vi "Periodic Tasks.vi"(8 "error in":errorcluster) -> ()   [LabVIEW 2016]
doc: "This VI runs in parallel to other tasks. It can contain as many user-defined periodic loops as you need. These can carry out PID or other sorts of timed response."
uses:
  <vilib>/Rock Robotics/WPI/DriverStation/WPI_DriverStationRobotMode2.ctl
  Robot Global Data.vi
  <vilib>/Rock Robotics/Network Tables/NT Write Boolean.vi
  <vilib>/Rock Robotics/Network Tables/NT Write Number.vi
  <vilib>/Rock Robotics/Network Tables/NT Read String.vi
  <vilib>/Rock Robotics/Network Tables/NT Write String.vi
  <vilib>/Rock Robotics/Network Tables/NT Read Number.vi
  <vilib>/Rock Robotics/WPI/Utilities/WPI_GetSetVariantRefNum.vi
  <vilib>/Rock Robotics/Network Tables/NT Read Numeric Array.vi
  <vilib>/Rock Robotics/Network Tables/NT Read Boolean.vi
  <vilib>/Rock Robotics/Network Tables/NT Write Numeric Array.vi
panel:
  in  "milliseconds to wait":u32=20
  out "Averaged Values 2":dbl(graph)
  out "Channel 1":dbl(graph)
  out "Channel 0":dbl(graph)
  in  "Range":dbl=100.0 format="%#_13g"
  out "Averaged Values":dbl(graph)=25.833333333333332
  out "<5?":i16(graph)=1
  out "Image Width":dbl(graph)=26.0
  in  "Past array Width":dbl[](array[numeric])=[26.0, 26.0, 26.0, 25.0, 26.0, 26.0]
  out "Gear Orient":bool=TRUE
  out "Gear In":bool=TRUE
  out "1 Width":dbl=17.0
  out "1 Height":dbl=26.0
  out "2 Width":dbl=8.5
  out "2 Height":dbl=13.0
  in  "Past array":dbl[](array[numeric])=[-10.0, -10.0, -10.0]
  in  "Lcal Pixy Out":dbl=-10.0
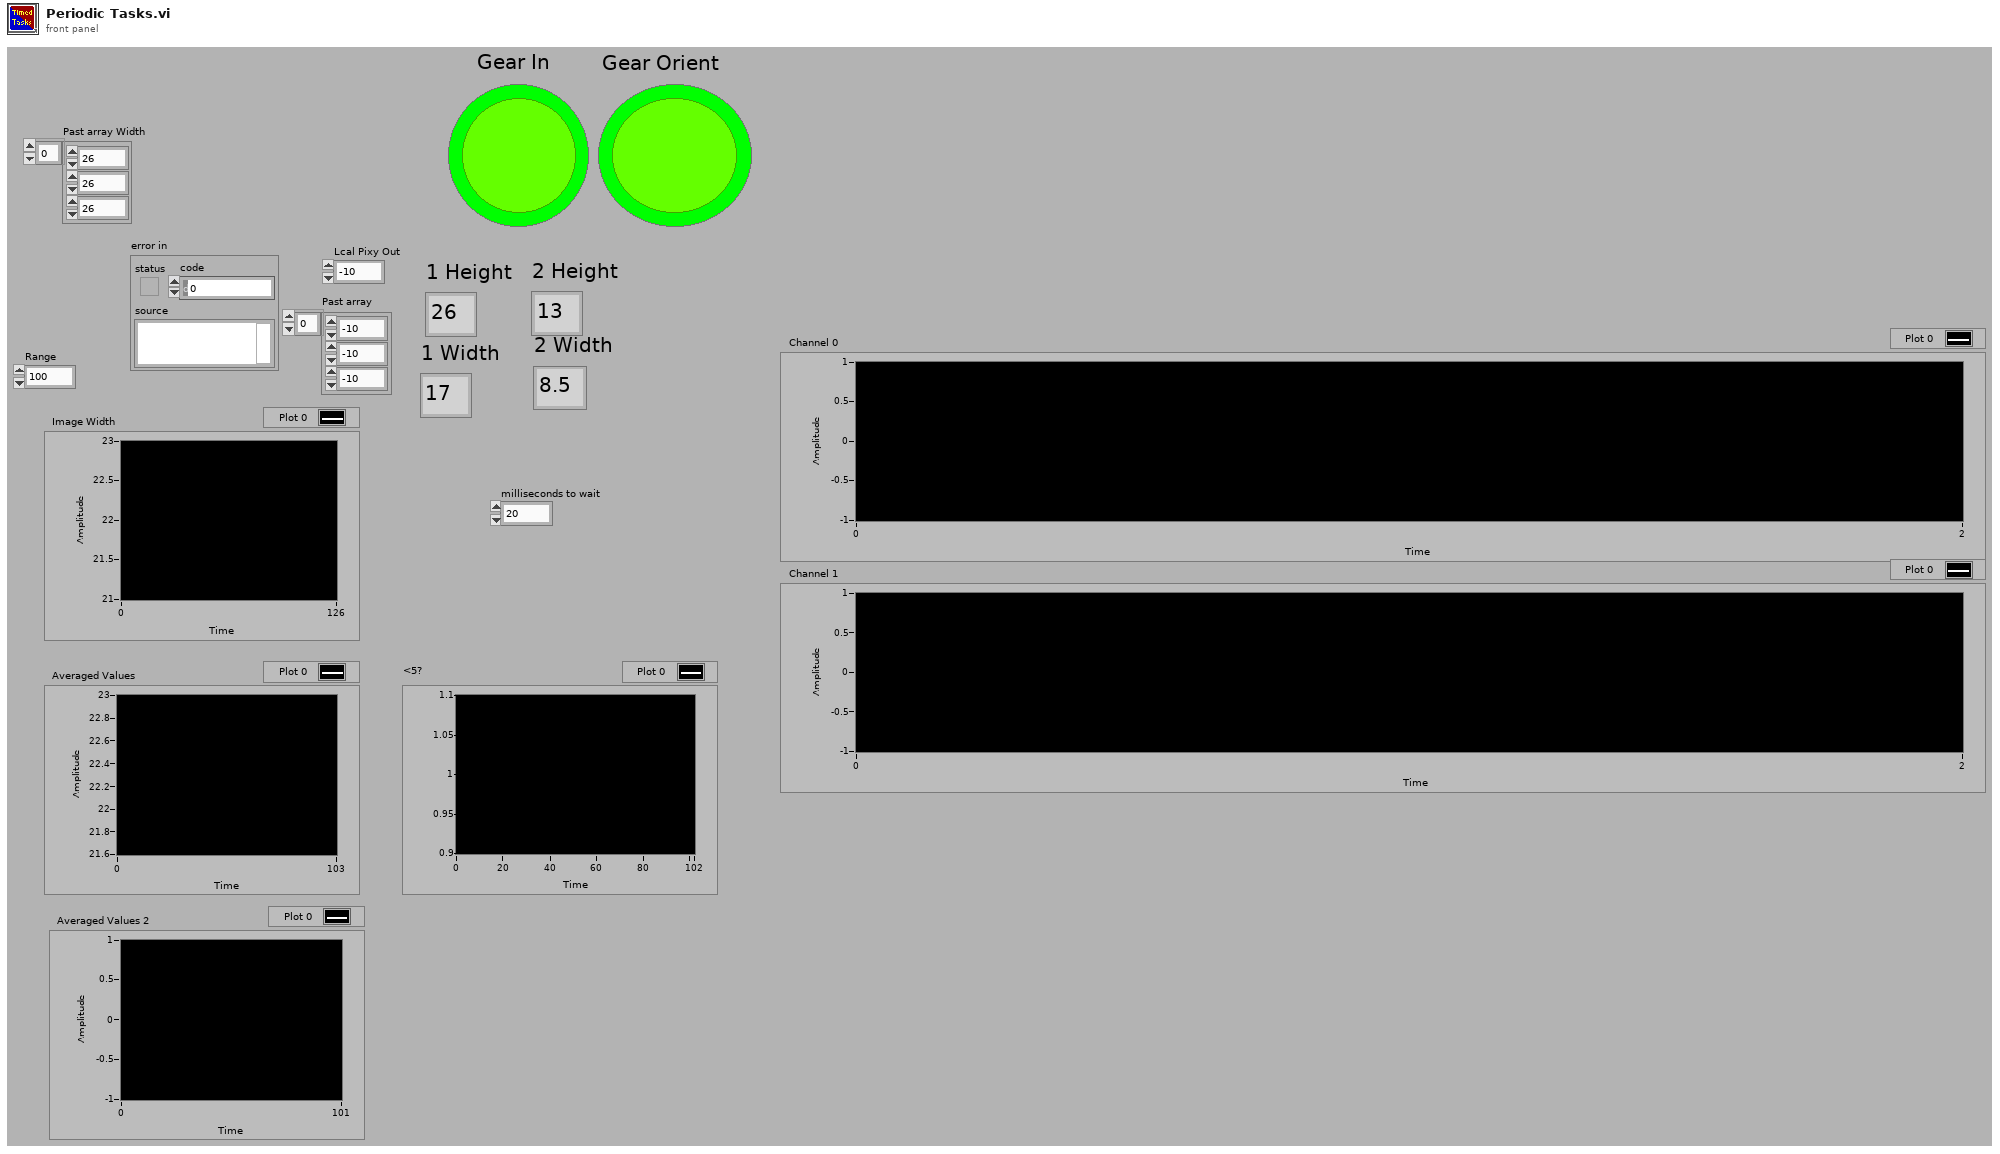
[diagram p1: front panel]
types:
  T1 = typedef "WPI_SwitchDevRef.ctl" = cluster{"DevStatus":errorcluster, "DIO Channel":T2, "CntIndex":T3, "Normally Closed":bool}
  T2 = typedef "FPGA_DIOChannel.ctl" = enum8{"DIO 0", "DIO 1", "DIO 2", "DIO 3", "DIO 4", "DIO 5", "DIO 6", "DIO 7", "DIO 8", "DIO 9", "DIO MXP 0", "DIO MXP 1", "DIO MXP 2", "DIO MXP 3", "DIO MXP 4", "DIO MXP 5", "DIO MXP 6", "DIO MXP 7", "DIO MXP 8", "DIO MXP 9", "DIO MXP 10", "DIO MXP 11", "DIO MXP 12", "DIO MXP 13", "DIO MXP 14", "DIO MXP 15", "SPI Port CS1", "SPI Port CS2", "SPI Port CS3", "SPI Port MISO", "SPI Port MOSI", "Invalid"}
  T3 = typedef "FPGA_CounterCtrSystemIndex.ctl" = enum8{"Ctr 0", "Ctr 1", "Ctr 2", "Ctr 3", "Ctr 4", "Ctr 5", "Ctr 6", "Ctr 7", "Invalid"}
  T4 = typedef "WPI_ServoDeviceRef.ctl" = cluster{"DeviceStatus":errorcluster, "PWM Channel":T5, "DeadBand":T6}
  T5 = typedef "FPGA_DIOPWMChannel.ctl" = enum8{"PWM 0", "PWM 1", "PWM 2", "PWM 3", "PWM 4", "PWM 5", "PWM 6", "PWM 7", "PWM 8", "PWM 9", "PWM MXP 0", "PWM MXP 1", "PWM MXP 2", "PWM MXP 3", "PWM MXP 4", "PWM MXP 5", "PWM MXP 6", "PWM MXP 7", "PWM MXP 8", "PWM MXP 9", "Invalid"}
  T6 = typedef "WPI_PWMDeadband.ctl" = cluster{"Name":string, "maxPositivePwm":i32, "minPositivePwm":i32, "centerPwm":i32, "maxNegativePwm":i32, "minNegativePwm":i32, "angularRange":u16}
  T7 = typedef "WPI_CounterDevRef.ctl" = cluster{"DevStatus":errorcluster, "CntIndex":T3}
  T8 = typedef "WPI_JoystickDevRef.ctl" = cluster{"Device":T9}
  T9 = typedef "WPI_JoystickDeviceEnum.ctl" = enum16{"USB 0", "USB 1", "USB 2", "USB 3", "USB 4", "USB 5"}
  T10 = typedef "WPI_DriverStationRobotMode2.ctl" = enum16{"Autonomous Disabled", "Autonomous Enabled", "Teleop Disabled", "Teleop Enabled", "Disconnected", "Finish", "Test Disabled", "Test Enabled", "Emergency Stopped"}
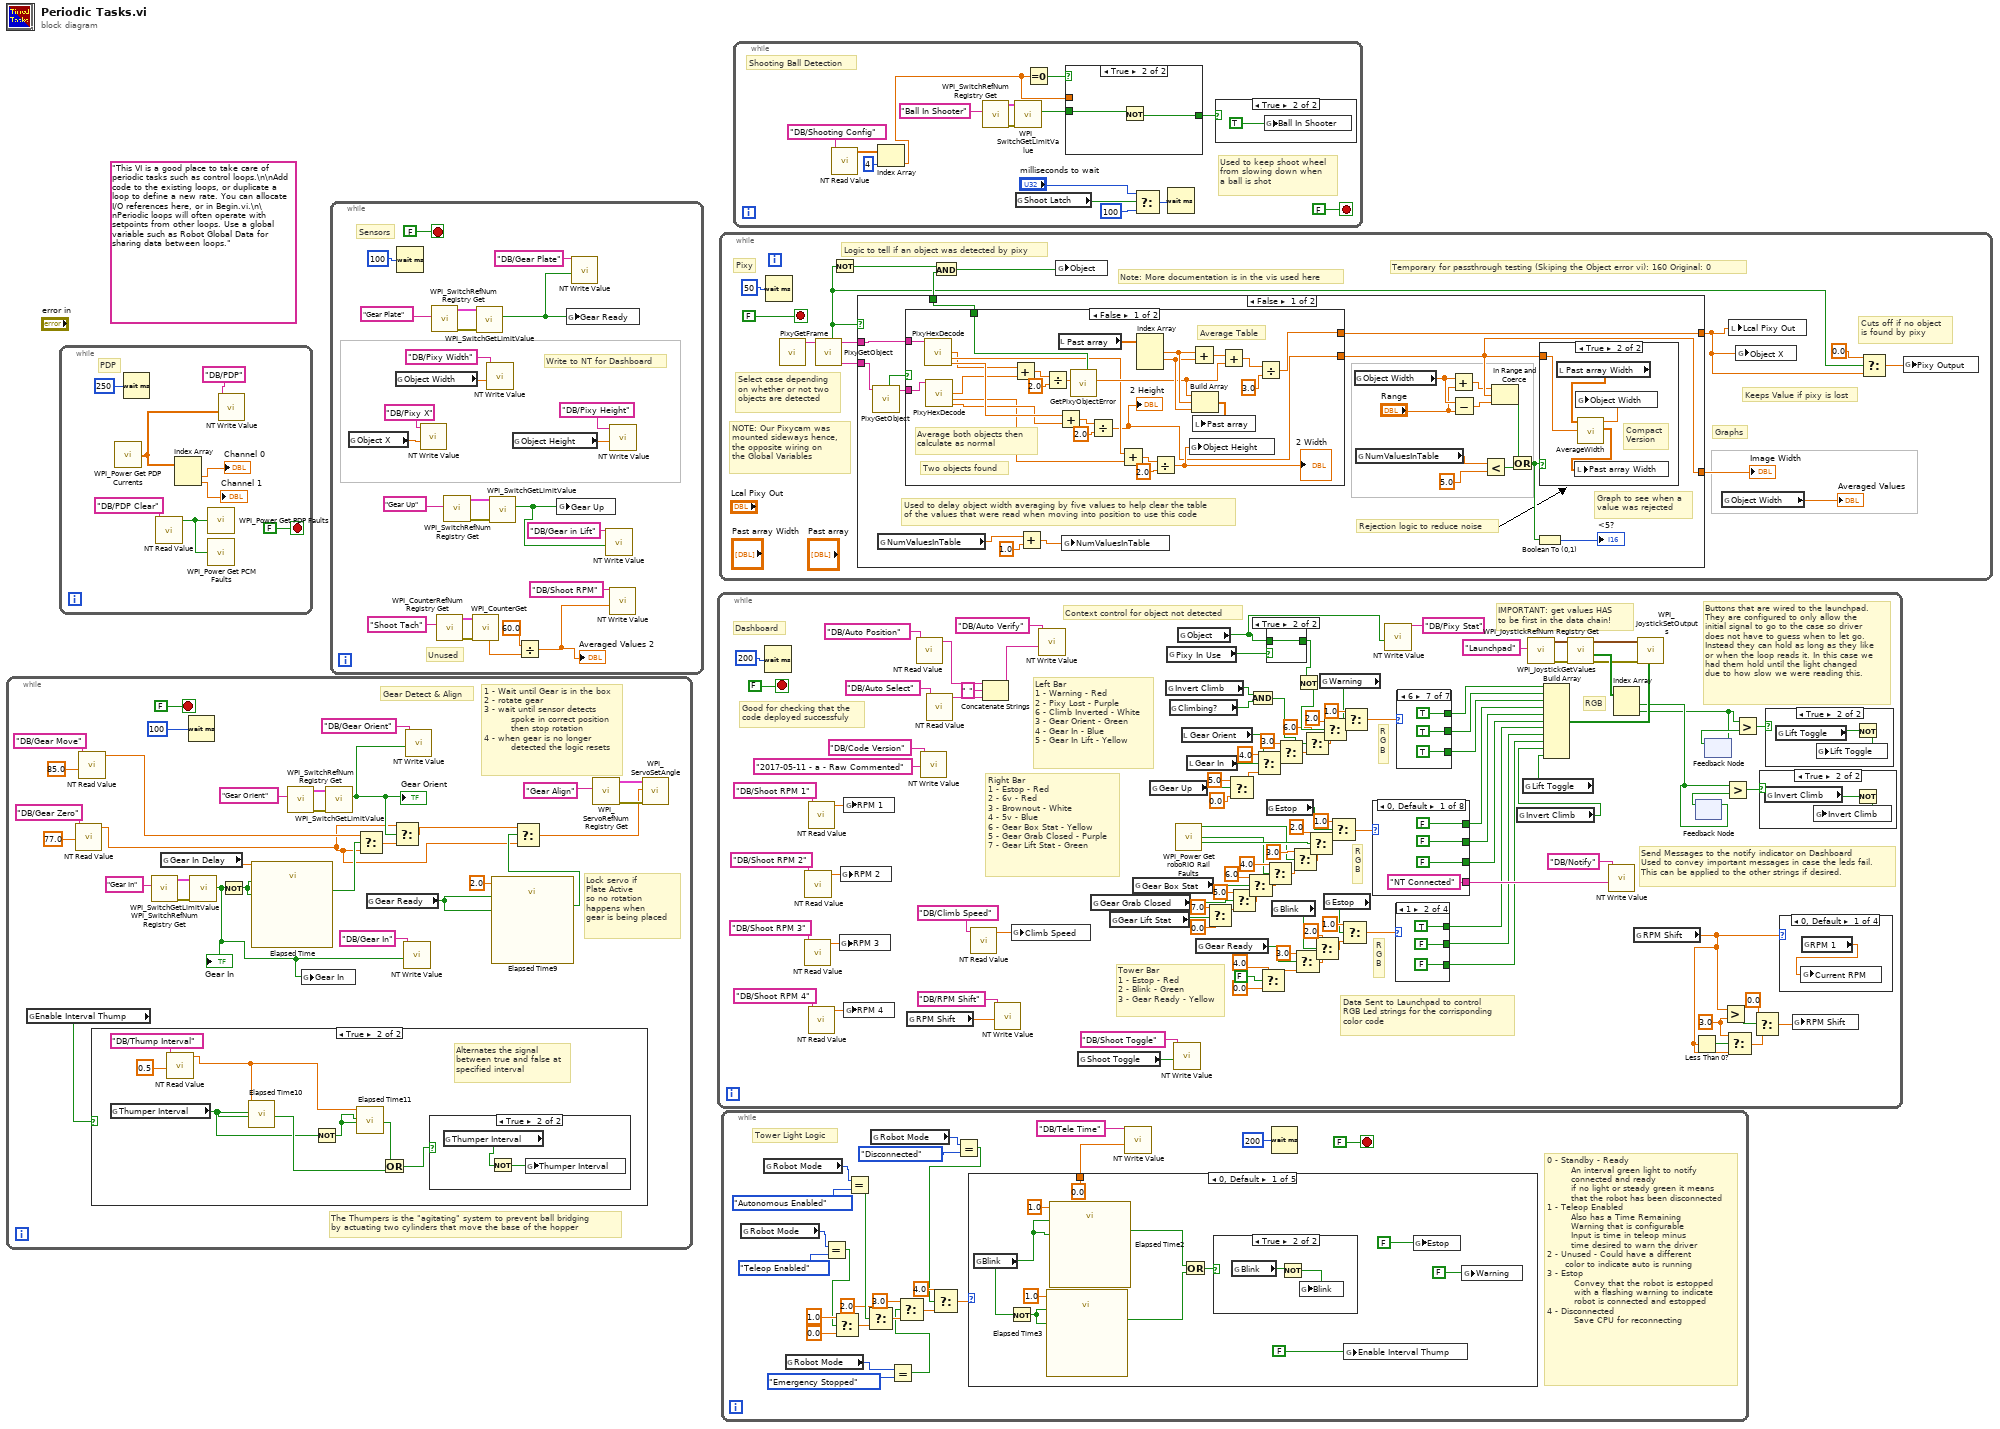
[diagram p0: block diagram]
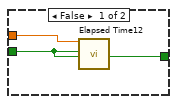
[diagram p2: hidden frame]
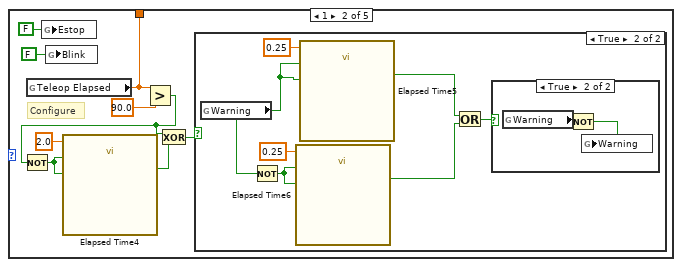
[diagram p5: hidden frame]
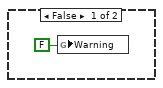
[diagram p6: hidden frame]
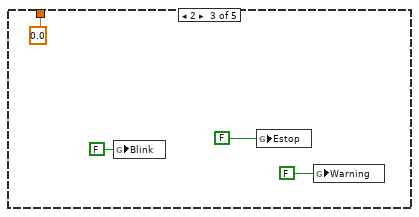
[diagram p8: hidden frame]
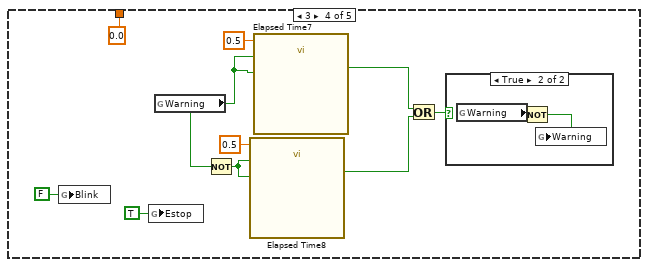
[diagram p9: hidden frame]
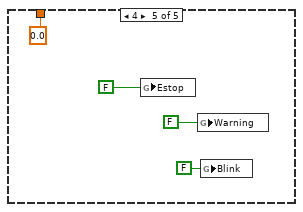
[diagram p11: hidden frame]
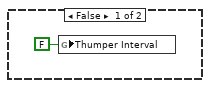
[diagram p12: hidden frame]
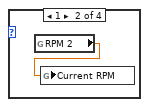
[diagram p14: hidden frame]
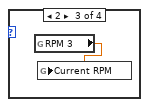
[diagram p15: hidden frame]
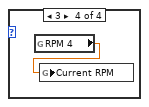
[diagram p16: hidden frame]
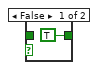
[diagram p19: hidden frame]
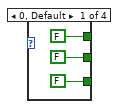
[diagram p20: hidden frame]
diagram:
  (unwired) "This VI is a good place to take care of periodic tasks such as control loops.\n\nAdd code to the existing loops, or duplicate a loop to define a new rate. You can allocate I/O references here, or in Begin.vi.\n\nPeriodic loops will often operate with setpoints from other loops. Use a global variable such as Robot Global Data for sharing data between loops."
  n1 = while {
    stop <- FALSE stop-if-true
    # "1 - Wait until Gear is in the box\n2 - rotate gear \n3 - wait until sensor detects \n         spoke in correct position\n         then stop rotation\n4 - when gear is no longer \n         detected the logic resets"
    # "The Thumpers is the \"agitating\" system to prevent ball bridging \nby actuating two cylinders that move the base of the hopper"
    # "Lock servo if\nPlate Active\nso no rotation\nhappens when\ngear is being placed"
    # "Gear Detect & Align"
    n2 = global read "Robot Global Data.vi" "Enable Interval Thump"() -> (w1:bool)
    n3 = call-poly <vilib>:"NT Read Value.vi"("Default Value"=77.0, "Name"="DB/Gear Zero") -> ("Numeric"=w3:dbl)  [unwired: 8 in, 1 out]
    n4 = call-poly <vilib>:"NT Read Value.vi"("Default Value"=85.0, "Name"="DB/Gear Move") -> ("Numeric"=w11:dbl)  [unwired: 8 in, 1 out]
    n5 = case shown="True" w1 {
      frame False {
        n6 = global write "Robot Global Data.vi" "Thumper Interval"(FALSE ("Thumper Interval")) -> ()
      }
      frame True {
        # "Alternates the signal\nbetween true and false at\nspecified interval"
        n7 = global read "Robot Global Data.vi" "Thumper Interval"() -> (w36:bool)
        n8 = call-poly <vilib>:"NT Read Value.vi"("Default Value"=0.5, "Name"="DB/Thump Interval") -> ("Numeric"=w33:dbl)  [unwired: 8 in, 1 out]
        n9 = call "Elapsed Time10"("Time Target (s)"=w33, "Reset"=w36, "Auto Reset"=w36) -> ("Time has Elapsed"=w38:bool)  [unwired: 9 in, 7 out]
        n10 = Not(x=w36) -> (.not. x?=w40:bool)
        n11 = call "Elapsed Time11"("Time Target (s)"=w33, "Reset"=w40, "Auto Reset"=w40) -> ("Time has Elapsed"=w39:bool)  [unwired: 9 in, 7 out]
        n12 = Or(x=w39, y=w38) -> (x .or. y?=w37:bool)
        n13 = case shown="True" w37 {
          frame False {
          }
          frame True {
            n14 = global read "Robot Global Data.vi" "Thumper Interval"() -> (w42:bool)
            n15 = Not(x=w42) -> (.not. x?=w41:bool)
            n16 = global write "Robot Global Data.vi" "Thumper Interval"(w41) -> ()
          }
        }
      }
    }
    n17 = call <vilib>:"WPI_SwitchRefNum Registry Get.vi"("refnum name"="Gear In") -> ("error out"=w28:errorcluster, "SwitchDevRef"=w29:T1)  [unwired: 9 in]
    n18 = global read "Robot Global Data.vi" "Gear In Delay"() -> (w21:dbl)
    n19 = Wait (ms)(milliseconds to wait=u32 100) -> ()  [unwired: 1 out]
    n20 = call <vilib>:"WPI_SwitchGetLimitValue.vi"("error in (no error)"=w28, "SwitchDevRef"=w29) -> ("Switch Pressed"=w2:bool)  [unwired: 7 in, 2 out]
    "Gear In" <- w2
    n21 = Not(x=w2) -> (.not. x?=w22:bool)
    n22 = call "Elapsed Time"("Time Target (s)"=w21, "Reset"=w22, "Auto Reset"=w22) -> ("Time has Elapsed"=w16:bool)  [unwired: 9 in, 7 out]
    n23 = call <vilib>:"WPI_SwitchRefNum Registry Get.vi"("refnum name"="Gear Orient") -> ("error out"=w24:errorcluster, "SwitchDevRef"=w25:T1)  [unwired: 9 in]
    n24 = global write "Robot Global Data.vi" "Gear In"(w2) -> ()
    n25 = call <vilib>:"WPI_SwitchGetLimitValue.vi"("error in (no error)"=w24, "SwitchDevRef"=w25) -> ("Switch Pressed"=w14:bool)  [unwired: 7 in, 2 out]
    "Gear Orient" <- w14
    n26 = Select(t=w11, s=w16, f=w3) -> (s? t:f=w26:dbl)
    n27 = global read "Robot Global Data.vi" "Gear Ready"() -> (w7:bool)
    n28 = Select(t=w3, s=w14, f=w26) -> (s? t:f=w4:dbl)
    n29 = call-poly <vilib>:"NT Write Value.vi"("Boolean"=w2, "Name"="DB/Gear In") -> ()  [unwired: 9 in, 1 out]
    n30 = call-poly <vilib>:"NT Write Value.vi"("Boolean"=w14, "Name"="DB/Gear Orient") -> ()  [unwired: 9 in, 1 out]
    n31 = call "Elapsed Time9"("Time Target (s)"=2.0, "Reset"=w7, "Auto Reset"=w7) -> ("Time has Elapsed"=w5:bool)  [unwired: 9 in, 7 out]
    n32 = Select(t=w4, s=w5, f=w3) -> (s? t:f=w8:dbl)
    n33 = call <vilib>:"WPI_ServoRefNum Registry Get.vi"("refnum name"="Gear Align") -> ("error out"=w17:errorcluster, "ServoDeviceRef"=w18:T4)  [unwired: 9 in]
    n34 = call <vilib>:"WPI_ServoSetAngle.vi"("error in (no error)"=w17, "Angle"=w8, "ServoDeviceRef"=w18) -> ()  [unwired: 7 in, 2 out]
  }
  n35 = while {
    stop <- FALSE stop-if-true
    # "PDP"
    n36 = call <vilib>:"WPI_Power Get PDP Currents.vi"() -> ("all currents (A)"=w45:dbl[])  [unwired: 13 in, 2 out]
    n37 = Wait (ms)(milliseconds to wait=u32 250) -> ()  [unwired: 1 out]
    n38 = call-poly <vilib>:"NT Read Value.vi"("Name"="DB/PDP Clear") -> ("Boolean"=w46:bool)  [unwired: 9 in, 1 out]
    n39 = Index Array(array=w45) -> (element #1=→"Channel 0":dbl, element #2=→"Channel 1":dbl)  [unwired: 2 in]
    n40 = call <vilib>:"WPI_Power Get PDP Faults.vi"("Clear Sticky Faults"=w46) -> ()  [unwired: 10 in, 5 out]
    n41 = call <vilib>:"WPI_Power Get PCM Faults.vi"("Clear Sticky Faults"=w46) -> ()  [unwired: 11 in, 4 out]
    n42 = call-poly <vilib>:"NT Write Value.vi"("Numeric Array"=w45, "Name"="DB/PDP") -> ()  [unwired: 9 in, 1 out]
  }
  n43 = while {
    stop <- FALSE stop-if-true
    # "Write to NT for Dashboard"
    # "Unused"
    # "Sensors"
    n44 = global read "Robot Global Data.vi" "Object X"() -> (w63:dbl)
    n45 = global read "Robot Global Data.vi" "Object Width"() -> (w65:dbl)
    n46 = Wait (ms)(milliseconds to wait=u32 100) -> ()  [unwired: 1 out]
    n47 = call-poly <vilib>:"NT Write Value.vi"("Numeric"=w63, "Name"="DB/Pixy X") -> ()  [unwired: 9 in, 1 out]
    n48 = call <vilib>:"WPI_SwitchRefNum Registry Get.vi"("refnum name"="Gear Plate") -> ("error out"=w73:errorcluster, "SwitchDevRef"=w72:T1)  [unwired: 9 in]
    n49 = call <vilib>:"WPI_CounterRefNum Registry Get.vi"("refnum name"="Shoot Tach") -> ("error out"=w54:errorcluster, "CounterDevRef"=w55:T7)  [unwired: 9 in]
    n50 = call <vilib>:"WPI_SwitchRefNum Registry Get.vi"("refnum name"="Gear Up") -> ("error out"=w62:errorcluster, "SwitchDevRef"=w61:T1)  [unwired: 9 in]
    n51 = call <vilib>:"WPI_CounterGet.vi"("error in (no error)"=w54, "CounterDevRef in"=w55) -> ("Period (sec)"=w57:dbl)  [unwired: 4 in, 5 out]
    n52 = call <vilib>:"WPI_SwitchGetLimitValue.vi"("error in (no error)"=w73, "SwitchDevRef"=w72) -> ("Switch Pressed"=w69:bool)  [unwired: 7 in, 2 out]
    n53 = call-poly <vilib>:"NT Write Value.vi"("Numeric"=w65, "Name"="DB/Pixy Width") -> ()  [unwired: 9 in, 1 out]
    n54 = call <vilib>:"WPI_SwitchGetLimitValue.vi"("error in (no error)"=w62, "SwitchDevRef"=w61) -> ("Switch Pressed"=w58:bool)  [unwired: 7 in, 2 out]
    n55 = global read "Robot Global Data.vi" "Object Height"() -> (w64:dbl)
    n56 = Divide(x=60.0, y=w57) -> (x/y=w51:dbl)
    "Averaged Values 2" <- w51
    n57 = global write "Robot Global Data.vi" "Gear Up"(w58) -> ()
    n58 = global write "Robot Global Data.vi" "Gear Ready"(w69) -> ()
    n59 = call-poly <vilib>:"NT Write Value.vi"("Boolean"=w69, "Name"="DB/Gear Plate") -> ()  [unwired: 9 in, 1 out]
    n60 = call-poly <vilib>:"NT Write Value.vi"("Boolean"=w58, "Name"="DB/Gear in Lift") -> ()  [unwired: 9 in, 1 out]
    n61 = call-poly <vilib>:"NT Write Value.vi"("Numeric"=w51, "Name"="DB/Shoot RPM") -> ()  [unwired: 9 in, 1 out]
    n62 = call-poly <vilib>:"NT Write Value.vi"("Numeric"=w64, "Name"="DB/Pixy Height") -> ()  [unwired: 9 in, 1 out]
  }
  n63 = while {
    stop <- FALSE stop-if-true
    w102 = 3.0 ("y")
    # "Good for checking that the\ncode deployed successfuly"
    # "IMPORTANT: get values HAS \nto be first in the data chain!"
    # "Buttons that are wired to the launchpad.\nThey are configured to only allow the \ninitial signal to go to the case so driver\ndoes not have to guess when to let go.\nInstead they can hold as long as they like\nor when the loop reads it. In this case we\nhad them hold until the light changed \ndue to how slow we were reading this."
    # "Context control for object not detected"
    # "Send Messages to the notify indicator on Dashboard\nUsed to convey important messages in case the leds fail.\nThis can be applied to the other strings if desired."
    # "R\nG\nB"
    # "R\nG\nB"
    # "R\nG\nB"
    # "Data Sent to Launchpad to control\nRGB Led strings for the corrisponding \ncolor code"
    # "Left Bar\n1 - Warning - Red\n2 - Pixy Lost - Purple \n6 - Climb Inverted - White\n3 - Gear Orient - Green\n4 - Gear In - Blue\n5 - Gear In Lift - Yellow"
    # "RGB"
    # "Tower Bar\n1 - Estop - Red\n2 - Blink - Green\n3 - Gear Ready - Yellow"
    # "Right Bar\n1 - Estop - Red\n2 - 6v - Red\n3 - Brownout - White\n4 - 5v - Blue\n6 - Gear Box Stat - Yellow\n5 - Gear Grab Closed - Purple\n7 - Gear Lift Stat - Green"
    # "Dashboard"
    n64 = Wait (ms)(milliseconds to wait=u32 200) -> ()  [unwired: 1 out]
    n65 = call-poly <vilib>:"NT Read Value.vi"("Name"="DB/Shoot RPM 3") -> ("Numeric"=w174:dbl)  [unwired: 9 in, 1 out]
    n66 = call-poly <vilib>:"NT Read Value.vi"("Name"="DB/Shoot RPM 2") -> ("Numeric"=w176:dbl)  [unwired: 9 in, 1 out]
    n67 = call-poly <vilib>:"NT Read Value.vi"("Name"="DB/Shoot RPM 1") -> ("Numeric"=w180:dbl)  [unwired: 9 in, 1 out]
    n68 = call-poly <vilib>:"NT Read Value.vi"("Name"="DB/Shoot RPM 4") -> ("Numeric"=w172:dbl)  [unwired: 9 in, 1 out]
    n69 = global write "Robot Global Data.vi" "RPM 3"(w174) -> ()
    n70 = global write "Robot Global Data.vi" "RPM 2"(w176) -> ()
    n71 = global write "Robot Global Data.vi" "RPM 1"(w180) -> ()
    n72 = global write "Robot Global Data.vi" "RPM 4"(w172) -> ()
    n73 = global read "Robot Global Data.vi" "RPM Shift"() -> (w170:dbl)
    n74 = call-poly <vilib>:"NT Read Value.vi"("Name"="DB/Auto Position") -> ("String"=w190:string)  [unwired: 9 in, 1 out]
    n75 = call-poly <vilib>:"NT Write Value.vi"("String"="2017-05-11 - a - Raw Commented", "Name"="DB/Code Version") -> ()  [unwired: 9 in, 1 out]
    n76 = call-poly <vilib>:"NT Read Value.vi"("Name"="DB/Auto Select") -> ("String"=w191:string)  [unwired: 9 in, 1 out]
    n77 = call-poly <vilib>:"NT Read Value.vi"("Name"="DB/Climb Speed") -> ("Numeric"=w178:dbl)  [unwired: 9 in, 1 out]
    n78 = Concatenate Strings(w190, " " ("string"), w191) -> (w189:string)
    n79 = call-poly <vilib>:"NT Write Value.vi"("Numeric"=w170, "Name"="DB/RPM Shift") -> ()  [unwired: 9 in, 1 out]
    n80 = global write "Robot Global Data.vi" "Climb Speed"(w178) -> ()
    n81 = call-poly <vilib>:"NT Write Value.vi"("String"=w189, "Name"="DB/Auto Verify") -> ()  [unwired: 9 in, 1 out]
    n82 = global read "Robot Global Data.vi" "Shoot Toggle"() -> (w90:bool)
    n83 = global read "Robot Global Data.vi" "Gear Grab Closed"() -> (w83:bool)
    n84 = global read "Robot Global Data.vi" "Gear Lift Stat"() -> (w92:bool)
    n85 = global read "Robot Global Data.vi" "Gear Box Stat"() -> (w84:bool)
    n86 = global read "Robot Global Data.vi" "Gear Up"() -> (w87:bool)
    n87 = global read "Robot Global Data.vi" "Invert Climb"() -> (w78:bool)
    n88 = global read "Robot Global Data.vi" "Pixy In Use"() -> (w120:bool)
    n89 = global read "Robot Global Data.vi" "Climbing?"() -> (w77:bool)
    n90 = call-poly <vilib>:"NT Write Value.vi"("Boolean"=w90, "Name"="DB/Shoot Toggle") -> ()  [unwired: 9 in, 1 out]
    n91 = call <vilib>:"WPI_Power Get roboRIO Rail Faults.vi"() -> ("Input Voltage Brown Out"=w144:bool, "5 V User Rail Short"=w145:bool, "6 V User Rail Short"=w146:bool)  [unwired: 10 in, 3 out]
    n92 = global read "Robot Global Data.vi" "Object"() -> (w114:bool)
    n93 = local read "Gear Orient"() -> (w122:bool)
    n94 = local read "Gear In"() -> (w121:bool)
    n95 = global read "Robot Global Data.vi" "Gear Ready"() -> (w124:bool)
    n96 = Select(t=7.0, s=w92, f=0.0) -> (s? t:f=w95:dbl)
    n97 = Select(t=5.0, s=w87, f=0.0) -> (s? t:f=w88:dbl)
    n98 = Select(t=5.0, s=w83, f=w95) -> (s? t:f=w147:dbl)
    n99 = Select(t=6.0, s=w84, f=w147) -> (s? t:f=w148:dbl)
    n100 = And(x=w78, y=w77) -> (x .and. y?=w76:bool)
    n101 = Select(t=4.0, s=w121, f=w88) -> (s? t:f=w163:dbl)
    n102 = Select(t=4.0, s=FALSE, f=0.0) -> (s? t:f=w133:dbl)
    n103 = case shown="True" w120 {
      tunnel: [TRUE ("Object") w203] -> w118
      tunnel: w114 -> [_ w203]
      frame False {
      }
      frame True {
      }
    }
    n104 = global read "Robot Global Data.vi" "Estop"() -> (w150:bool)
    n105 = Select(t=4.0, s=w145, f=w148) -> (s? t:f=w155:dbl)
    n106 = global read "Robot Global Data.vi" "Blink"() -> (w125:bool)
    n107 = Select(t=3.0, s=w122, f=w163) -> (s? t:f=w79:dbl)
    n108 = Select(t=3.0, s=w144, f=w155) -> (s? t:f=w156:dbl)
    n109 = Select(t=3.0, s=w124, f=w133) -> (s? t:f=w134:dbl)
    n110 = Not(x=w118) -> (.not. x?=w119:bool)
    n111 = Select(t=6.0, s=w76, f=w79) -> (s? t:f=w81:dbl)
    n112 = Select(t=2.0, s=w146, f=w156) -> (s? t:f=w157:dbl)
    n113 = Select(t=2.0, s=w125, f=w134) -> (s? t:f=w135:dbl)
    n114 = global read "Robot Global Data.vi" "Warning"() -> (w137:bool)
    n115 = Select(t=2.0, s=w119, f=w81) -> (s? t:f=w167:dbl)
    n116 = global read "Robot Global Data.vi" "Estop"() -> (w126:bool)
    n117 = Select(t=1.0, s=w150, f=w157) -> (s? t:f=w151:dbl)
    n118 = Select(t=1.0, s=w126, f=w135) -> (s? t:f=w136:dbl)
    n119 = Select(t=1.0, s=w137, f=w167) -> (s? t:f=w168:dbl)
    n120 = case shown="0, Default" w151 {
      tunnel: [FALSE TRUE TRUE TRUE FALSE TRUE TRUE FALSE] -> w140
      tunnel: [FALSE FALSE FALSE TRUE FALSE FALSE TRUE TRUE] -> w139
      tunnel: [FALSE FALSE FALSE TRUE TRUE TRUE FALSE FALSE] -> w138
      tunnel: ["NT Connected" ("String") "EStop - Reset Rio" ("String") "6v Rail Short" ("String") "Brownout" ("String") "5v Rail Short" ("String") "NT Connected" ("String") "NT Connected" ("String") "NT Connected" ("String")] -> w158
      frame 0, Default {
      }
      frame 1 {
      }
      frame 2 {
      }
      frame 3 {
      }
      frame 4 {
      }
      frame 5 {
      }
      frame 6 {
      }
      frame 7 {
      }
    }
    n121 = call-poly <vilib>:"NT Write Value.vi"("Boolean"=w114, "Name"="DB/Pixy Stat") -> ()  [unwired: 9 in, 1 out]
    n122 = case shown="1" w136 {
      tunnel: [FALSE TRUE FALSE TRUE] -> w117
      tunnel: [FALSE FALSE TRUE TRUE] -> w116
      tunnel: [FALSE FALSE FALSE FALSE] -> w115
      frame 0, Default {
      }
      frame 1 {
      }
      frame 2 {
      }
      frame 3 {
      }
    }
    n123 = case shown="6" w168 {
      tunnel: [FALSE TRUE TRUE FALSE FALSE TRUE TRUE] -> w166
      tunnel: [FALSE FALSE FALSE TRUE FALSE TRUE TRUE] -> w165
      tunnel: [FALSE FALSE TRUE FALSE TRUE FALSE TRUE] -> w164
      frame 0, Default {
      }
      frame 1 {
      }
      frame 2 {
      }
      frame 3 {
      }
      frame 4 {
      }
      frame 5 {
      }
      frame 6 {
      }
    }
    n124 = global read "Robot Global Data.vi" "Invert Climb"() -> (w82:bool)
    n125 = global read "Robot Global Data.vi" "Lift Toggle"() -> (w89:bool)
    n126 = call <vilib>:"WPI_JoystickRefNum Registry Get.vi"("refnum name"="Launchpad") -> ("error out"=w101:errorcluster, "JoystickDevRef"=w100:T8)  [unwired: 9 in]
    n127 = Build Array(w166, w165, w164, w140, w139, w138, w117, w116, w115, w82, w89) -> (w141:bool[])
    n128 = call <vilib>:"WPI_JoystickGetValues.vi"("error in (no error)"=w101, "JoystickDevRef"=w100) -> ("error out"=w98:errorcluster, "Buttons"=w113:bool[], "JoystickDevRef"=w99:T8)  [unwired: 5 in, 2 out]
    n129 = call-poly <vilib>:"NT Write Value.vi"("String"=w158, "Name"="DB/Notify") -> ()  [unwired: 9 in, 1 out]
    n130 = Index Array(array=w113) -> (element #1=w97:bool, element #2=w96:bool)  [unwired: 2 in]
    n131 = global read "Robot Global Data.vi" "RPM Shift"() -> (w103:dbl)
    n132 = call <vilib>:"WPI_JoystickSetOutputs.vi"("Outputs"=w141, "error in (no error)"=w98, "JoystickDevRef"=w99) -> ()  [unwired: 7 in, 2 out]
    n133 = Less Than 0?(x=w103) -> (x < 0?=w106:bool)
    n134 = feedback #1() -> (w109:bool)  [unwired: 1 in]
    n135 = feedback-in #1(w97) -> ()
    n136 = feedback #2() -> (w111:bool)  [unwired: 1 in]
    n137 = feedback-in #2(w96) -> ()
    n138 = Greater?(x=w103, y=w102) -> (0:w105:bool)
    n139 = Greater?(x=w97, y=w109) -> (0:w110:bool)
    n140 = Select(t=w102, s=w106, f=w103) -> (s? t:f=w107:dbl)
    n141 = Greater?(x=w96, y=w111) -> (0:w112:bool)
    n142 = Select(t=0.0, s=w105, f=w107) -> (s? t:f=w108:dbl)
    n143 = case shown="True" w110 {
      frame False {
      }
      frame True {
        n144 = global read "Robot Global Data.vi" "Invert Climb"() -> (w199:bool)
        n145 = Not(x=w199) -> (.not. x?=w198:bool)
        n146 = global write "Robot Global Data.vi" "Invert Climb"(w198) -> ()
      }
    }
    n147 = case shown="True" w112 {
      frame False {
      }
      frame True {
        n148 = global read "Robot Global Data.vi" "Lift Toggle"() -> (w201:bool)
        n149 = Not(x=w201) -> (.not. x?=w200:bool)
        n150 = global write "Robot Global Data.vi" "Lift Toggle"(w200) -> ()
      }
    }
    n151 = case shown="0, Default" w103 {
      frame 0, Default {
        n152 = global read "Robot Global Data.vi" "RPM 1"() -> (w194:dbl)
        n153 = global write "Robot Global Data.vi" "Current RPM"(w194) -> ()
      }
      frame 1 {
        n154 = global read "Robot Global Data.vi" "RPM 2"() -> (w195:dbl)
        n155 = global write "Robot Global Data.vi" "Current RPM"(w195) -> ()
      }
      frame 2 {
        n156 = global read "Robot Global Data.vi" "RPM 3"() -> (w196:dbl)
        n157 = global write "Robot Global Data.vi" "Current RPM"(w196) -> ()
      }
      frame 3 {
        n158 = global read "Robot Global Data.vi" "RPM 4"() -> (w197:dbl)
        n159 = global write "Robot Global Data.vi" "Current RPM"(w197) -> ()
      }
    }
    n160 = global write "Robot Global Data.vi" "RPM Shift"(w108) -> ()
  }
  n161 = while {
    stop <- FALSE stop-if-true
    # "Note: More documentation is in the vis used here"
    # "NOTE: Our Pixycam was\nmounted sideways hence,\nthe opposite wiring on\nthe Global Variables"
    # "Keeps Value if pixy is lost"
    # "Cuts off if no object\nis found by pixy"
    # "Select case depending\non whether or not two\nobjects are detected"
    # "Graphs"
    # "Logic to tell if an object was detected by pixy"
    # "Temporary for passthrough testing (Skiping the Object error vi): 160 Original: 0"
    # "Pixy"
    n162 = Wait (ms)(milliseconds to wait=u32 50) -> ()  [unwired: 1 out]
    n163 = call "PixyGetFrame.vi"() -> ("Frame"=w277:string)  [unwired: 11 in]
    n164 = call "PixyGetObject.vi"("Input Frame"=w277) -> ("Remainder of Frame"=w276:string, "Object"=w275:string, "Empty?"=w273:bool)  [unwired: 8 in]
    n165 = Not(x=w273) -> (.not. x?=w279:bool)
    n166 = case shown="False" w273 {
      tunnel: [w302 w350] -> w271
      tunnel: w276 -> [w301 _]
      tunnel: w275 -> [w299 _]
      tunnel: [w297 FALSE] -> w274
      tunnel: [w291 w348] -> w270
      frame False {
        # "Used to delay object width averaging by five values to help clear the table\nof the values that were read when moving into position to use this code"
        # "Rejection logic to reduce noise"
        # "Graph to see when a \nvalue was rejected"
        n167 = call "PixyGetObject.vi"("Input Frame"=w301) -> ("Object"=w298:string, "Empty?"=w300:bool)  [unwired: 8 in, 1 out]
        n168 = global read "Robot Global Data.vi" "NumValuesInTable"() -> (w294:dbl)
        n169 = case shown="False" w300 {
          tunnel: [w327 w341] -> w302
          tunnel: w299 -> [w323 w338]
          tunnel: w298 -> [w322 _]
          tunnel: [w319 w337] -> w297
          tunnel: [w307 w334] -> w291
          frame False {
            # "Two objects found"
            # "Average both objects then\ncalculate as normal"
            # "Average Table"
            n170 = call "PixyHexDecode.vi"("Object"=w323) -> ("Y"=w309:dbl, "Width"=w312:dbl, "Height"=w314:dbl)  [unwired: 10 in, 2 out]
            n171 = call "PixyHexDecode.vi"("Object"=w322) -> ("Y"=w308:dbl, "Width"=w311:dbl, "Height"=w313:dbl)  [unwired: 10 in, 2 out]
            n172 = Add(x=w309, y=w308) -> (x+y=w325:dbl)
            n173 = Divide(x=w325, y=2.0) -> (x/y=w321:dbl)
            n174 = Add(x=w314, y=w313) -> (x+y=w318:dbl)
            n175 = local read "Past array"() -> (w333:dbl[])
            n176 = call "GetPixyObjectError.vi"("X Value"=w321) -> ("Output"=w320:dbl, "Object In Parameters"=w319:bool)  [unwired: 9 in]
            n177 = Divide(x=w318, y=2.0) -> (x/y=w307:dbl)
            "2 Height" <- w307
            n178 = Add(x=w312, y=w311) -> (x+y=w316:dbl)
            n179 = Index Array(array=w333) -> (element #1=w332:dbl, element #2=w331:dbl)  [unwired: 3 in, 1 out]
            n180 = Divide(x=w316, y=2.0) -> (x/y=w310:dbl)
            "2 Width" <- w310
            n181 = global write "Robot Global Data.vi" "Object Height"(w310) -> ()
            n182 = Add(x=w332, y=w331) -> (x+y=w330:dbl)
            n183 = Build Array(w320, w332, w331) -> (w326:dbl[])
            n184 = local write "Past array"(w326) -> ()
            n185 = Add(x=w330, y=w320) -> (x+y=w329:dbl)
            n186 = Divide(x=w329, y=3.0) -> (x/y=w327:dbl)
          }
          frame True {
            # "One Object found"
            # "Average Table"
            n187 = call "PixyHexDecode.vi"("Object"=w338) -> ("Y"=w335:dbl, "Width"=w336:dbl, "Height"=w334:dbl)  [unwired: 10 in, 2 out]
            "1 Width" <- w336
            "1 Height" <- w334
            n188 = call "GetPixyObjectError.vi"("X Value"=w335) -> ("Output"=w340:dbl, "Object In Parameters"=w337:bool)  [unwired: 9 in]
            n189 = global write "Robot Global Data.vi" "Object Height"(w336) -> ()
            n190 = local read "Past array"() -> (w347:dbl[])
            n191 = Index Array(array=w347) -> (element #1=w346:dbl, element #2=w345:dbl)  [unwired: 3 in, 1 out]
            n192 = Add(x=w346, y=w345) -> (x+y=w344:dbl)
            n193 = Build Array(w340, w346, w345) -> (w339:dbl[])
            n194 = Add(x=w344, y=w340) -> (x+y=w343:dbl)
            n195 = local write "Past array"(w339) -> ()
            n196 = Divide(x=w343, y=3.0) -> (x/y=w341:dbl)
          }
        }
        n197 = Add(x=w294, y=1.0) -> (x+y=w292:dbl)
        n198 = global write "Robot Global Data.vi" "NumValuesInTable"(w292) -> ()
        n199 = global read "Robot Global Data.vi" "Object Width"() -> (w290:dbl)
        n200 = global read "Robot Global Data.vi" "NumValuesInTable"() -> (w296:dbl)
        n201 = Add(x=w290, y="Range") -> (x+y=w287:dbl)
        n202 = Subtract(x=w290, y="Range") -> (x-y=w288:dbl)
        n203 = Less?(x=w296, y=5.0) -> (x < y?=w285:bool)
        n204 = In Range and Coerce(upper limit=w287, x=w291, lower limit=w288) -> (In Range?=w286:bool)  [unwired: 1 out]
        n205 = Or(x=w286, y=w285) -> (x .or. y?=w283:bool)
        n206 = Boolean To (0,1)(Boolean=w283) -> (0, 1=→"<5?":i16)
        n207 = case shown="True" w283 {
          tunnel: w291 -> [_ w305]
          frame False {
          }
          frame True {
            # "Compact\nVersion"
            n208 = local read "Past array Width"() -> (w304:dbl[])
            n209 = call "AverageWidth.vi"("Width"=w305, "Past array Width"=w304) -> ("Array"=w303:dbl[], "mean"=w306:dbl)  [unwired: 8 in]
            n210 = local write "Past array Width"(w303) -> ()
            n211 = global write "Robot Global Data.vi" "Object Width"(w306) -> ()
          }
        }
      }
      frame True {
        w348 = 0.0 ("Height")
        # "Keep Previous value when object is lost"
        # "Zero Variables"
        n212 = local read "Lcal Pixy Out"() -> (w350:dbl)
        n213 = global write "Robot Global Data.vi" "NumValuesInTable"(w348) -> ()
      }
    }
    "Image Width" <- w270
    n214 = And(x=w279, y=w274) -> (x .and. y?=w278:bool)
    n215 = global write "Robot Global Data.vi" "Object"(w278) -> ()
    n216 = global read "Robot Global Data.vi" "Object Width"() -> (→"Averaged Values":dbl)
    n217 = local write "Lcal Pixy Out"(w271) -> ()
    n218 = global write "Robot Global Data.vi" "Object X"(w271) -> ()
    n219 = Select(t=0.0, s=w273, f=w271) -> (s? t:f=w272:dbl)
    n220 = global write "Robot Global Data.vi" "Pixy Output"(w272) -> ()
  }
  n221 = while {
    stop <- FALSE stop-if-true
    # "0 - Standby - Ready\n        An interval green light to notify\n        connected and ready\n        if no light or steady green it means\n        that the robot has been disconnected\n1 - Teleop Enabled\n        Also has a Time Remaining\n        Warning that is configurable\n        Input is time in teleop minus \n        time desired to warn the driver\n2 - Unused - Could have a different\n      color to indicate auto is running\n3 - Estop\n         Convey that the robot is estopped\n         with a flashing warning to indicate\n         robot is connected and estopped\n4 - Disconnected\n         Save CPU for reconnecting"
    # "Tower Light Logic"
    n222 = global read "Robot Global Data.vi" "Robot Mode"() -> (w372:T10)
    n223 = global read "Robot Global Data.vi" "Robot Mode"() -> (w366:T10)
    n224 = global read "Robot Global Data.vi" "Robot Mode"() -> (w374:T10)
    n225 = Equal?(x=w372, y=WPI_DriverStationRobotMode2."Teleop Enabled") -> (x = y?=w362:bool)
    n226 = Select(t=1.0, s=w362, f=0.0) -> (s? t:f=w369:dbl)
    n227 = Equal?(x=w366, y=WPI_DriverStationRobotMode2."Autonomous Enabled") -> (x = y?=w364:bool)
    n228 = Select(t=2.0, s=w364, f=w369) -> (s? t:f=w361:dbl)
    n229 = global read "Robot Global Data.vi" "Robot Mode"() -> (w357:T10)
    n230 = Equal?(x=w374, y=WPI_DriverStationRobotMode2."Emergency Stopped") -> (x = y?=w358:bool)
    n231 = Select(t=3.0, s=w358, f=w361) -> (s? t:f=w359:dbl)
    n232 = Equal?(x=w357, y=WPI_DriverStationRobotMode2."Disconnected") -> (x = y?=w354:bool)
    n233 = Select(t=4.0, s=w354, f=w359) -> (s? t:f=w353:dbl)
    n234 = case shown="0, Default" w353 {
      tunnel: [0.0 ("Teleop Elapsed") w389 0.0 ("Teleop Elapsed") 0.0 ("Teleop Elapsed") 0.0 ("Teleop Elapsed")] -> w351
      frame 0, Default {
        n235 = global read "Robot Global Data.vi" "Blink"() -> (w380:bool)
        n236 = Not(x=w380) -> (.not. x?=w381:bool)
        n237 = call "Elapsed Time3"("Time Target (s)"=1.0, "Reset"=w381, "Auto Reset"=w381) -> ("Time has Elapsed"=w382:bool)  [unwired: 9 in, 7 out]
        n238 = call "Elapsed Time2"("Time Target (s)"=1.0, "Reset"=w380, "Auto Reset"=w380) -> ("Time has Elapsed"=w383:bool)  [unwired: 9 in, 7 out]
        n239 = Or(x=w383, y=w382) -> (x .or. y?=w384:bool)
        n240 = case shown="True" w384 {
          frame False {
          }
          frame True {
            n241 = global read "Robot Global Data.vi" "Blink"() -> (w388:bool)
            n242 = Not(x=w388) -> (.not. x?=w387:bool)
            n243 = global write "Robot Global Data.vi" "Blink"(w387) -> ()
          }
        }
        n244 = global write "Robot Global Data.vi" "Enable Interval Thump"(FALSE) -> ()
        n245 = global write "Robot Global Data.vi" "Estop"(FALSE ("Blink")) -> ()
        n246 = global write "Robot Global Data.vi" "Warning"(FALSE ("Blink")) -> ()
      }
      frame 1 {
        # "Configure"
        n247 = global read "Robot Global Data.vi" "Teleop Elapsed"() -> (w389:dbl)
        n248 = global write "Robot Global Data.vi" "Estop"(FALSE ("Blink")) -> ()
        n249 = global write "Robot Global Data.vi" "Blink"(FALSE ("Blink")) -> ()
        n250 = Greater?(x=w389, y=90.0) -> (0:w393:bool)
        n251 = Not(x=w393) -> (.not. x?=w396:bool)
        n252 = call "Elapsed Time4"("Time Target (s)"=2.0, "Reset"=w396, "Auto Reset"=w396) -> ("Time has Elapsed"=w391:bool)  [unwired: 9 in, 7 out]
        n253 = Exclusive Or(1:w391, 2:w393) -> (0:w392:bool)
        n254 = case shown="True" w392 {
          frame False {
            n255 = global write "Robot Global Data.vi" "Warning"(FALSE ("Blink")) -> ()
          }
          frame True {
            n256 = global read "Robot Global Data.vi" "Warning"() -> (w399:bool)
            n257 = Not(x=w399) -> (.not. x?=w400:bool)
            n258 = call "Elapsed Time6"("Time Target (s)"=0.25, "Reset"=w400, "Auto Reset"=w400) -> ("Time has Elapsed"=w401:bool)  [unwired: 9 in, 7 out]
            n259 = call "Elapsed Time5"("Time Target (s)"=0.25, "Reset"=w399, "Auto Reset"=w399) -> ("Time has Elapsed"=w402:bool)  [unwired: 9 in, 7 out]
            n260 = Or(x=w402, y=w401) -> (x .or. y?=w403:bool)
            n261 = case shown="True" w403 {
              frame False {
              }
              frame True {
                n262 = global read "Robot Global Data.vi" "Warning"() -> (w407:bool)
                n263 = Not(x=w407) -> (.not. x?=w406:bool)
                n264 = global write "Robot Global Data.vi" "Warning"(w406) -> ()
              }
            }
          }
        }
      }
      frame 2 {
        n265 = global write "Robot Global Data.vi" "Blink"(FALSE ("Blink")) -> ()
        n266 = global write "Robot Global Data.vi" "Estop"(FALSE ("Blink")) -> ()
        n267 = global write "Robot Global Data.vi" "Warning"(FALSE ("Blink")) -> ()
      }
      frame 3 {
        n268 = global write "Robot Global Data.vi" "Blink"(FALSE ("Blink")) -> ()
        n269 = global write "Robot Global Data.vi" "Estop"(TRUE ("Estop")) -> ()
        n270 = global read "Robot Global Data.vi" "Warning"() -> (w414:bool)
        n271 = Not(x=w414) -> (.not. x?=w416:bool)
        n272 = call "Elapsed Time8"("Time Target (s)"=0.5, "Reset"=w416, "Auto Reset"=w416) -> ("Time has Elapsed"=w417:bool)  [unwired: 9 in, 7 out]
        n273 = call "Elapsed Time7"("Time Target (s)"=0.5, "Reset"=w414, "Auto Reset"=w414) -> ("Time has Elapsed"=w418:bool)  [unwired: 9 in, 7 out]
        n274 = Or(x=w418, y=w417) -> (x .or. y?=w419:bool)
        n275 = case shown="True" w419 {
          frame False {
          }
          frame True {
            n276 = global read "Robot Global Data.vi" "Warning"() -> (w423:bool)
            n277 = Not(x=w423) -> (.not. x?=w422:bool)
            n278 = global write "Robot Global Data.vi" "Warning"(w422) -> ()
          }
        }
      }
      frame 4 {
        n279 = global write "Robot Global Data.vi" "Estop"(FALSE ("Blink")) -> ()
        n280 = global write "Robot Global Data.vi" "Warning"(FALSE ("Blink")) -> ()
        n281 = global write "Robot Global Data.vi" "Blink"(FALSE ("Blink")) -> ()
      }
    }
    n282 = call-poly <vilib>:"NT Write Value.vi"("Numeric"=w351, "Name"="DB/Tele Time") -> ()  [unwired: 9 in, 1 out]
    n283 = Wait (ms)(milliseconds to wait=u32 200) -> ()  [unwired: 1 out]
  }
  n284 = while {
    stop <- FALSE stop-if-true
    # "Used to keep shoot wheel\nfrom slowing down when\na ball is shot"
    # "Shooting Ball Detection"
    n285 = call-poly <vilib>:"NT Read Value.vi"("Name"="DB/Shooting Config") -> ("Numeric Array"=w436:dbl[])  [unwired: 9 in, 1 out]
    n286 = Index Array(array=w436, index=4) -> (element=w429:dbl)
    n287 = call <vilib>:"WPI_SwitchRefNum Registry Get.vi"("refnum name"="Ball In Shooter") -> ("error out"=w433:errorcluster, "SwitchDevRef"=w432:T1)  [unwired: 9 in]
    n288 = call <vilib>:"WPI_SwitchGetLimitValue.vi"("error in (no error)"=w433, "SwitchDevRef"=w432) -> ("Switch Pressed"=w428:bool)  [unwired: 7 in, 2 out]
    n289 = global read "Robot Global Data.vi" "Shoot Latch"() -> (w438:bool)
    n290 = Equal To 0?(x=w429) -> (x = 0?=w430:bool)
    n291 = case shown="True" w430 {
      tunnel: w428 -> [w445 w447]
      tunnel: [w444 w446] -> w431
      tunnel: w429 -> [w443 _]
      frame False {
        n292 = call "Elapsed Time12"("Time Target (s)"=w443, "Reset"=w445, "Auto Reset"=w445) -> ("Time has Elapsed"=w444:bool)  [unwired: 9 in, 7 out]
      }
      frame True {
        n293 = Not(x=w447) -> (.not. x?=w446:bool)
      }
    }
    n294 = Select(t="milliseconds to wait", s=w438, f=u32 100) -> (s? t:f=w440:u32)
    n295 = Wait (ms)(milliseconds to wait=w440) -> ()  [unwired: 1 out]
    n296 = case shown="True" w431 {
      frame False {
      }
      frame True {
        n297 = global write "Robot Global Data.vi" "Ball In Shooter"(TRUE) -> ()
      }
    }
  }
